vi "Sparger_syringe_rinsing_subVI_BM.vi"(4 "N syringe rinses":i32=3, 5 "COM Port":refnum<visa-resource-name>="COM12", 6 "N sparge rinses":i32=3, 7 "Pump Parameters":T1={"Speed 1"="150", "Speed 2"="250", "Speed 3"="450", "Speed 4"="250", "UW/Sample"="5", "Sparge"="2", "Std"="4", "Waste"="15", "Air"="14", "Milli-Q"="1", "H2SO4"="6", "NaOH"="3", "Catalyst"="7", "Cell (H+ side)"="8", "Cell (sample side)"="9", "NaCl"="11"}, 8 "Extra Milli-Q (ml)":dbl=2.0, 9 "step to ml":dbl=1920.0, 10 "Total Vol. (mL)":dbl=12.0, 11 "Sample Volume":dbl=10.0) -> ()   [LabVIEW 2021]
panel:
  out "Full Command":string="V450O1P38400O15D38400"
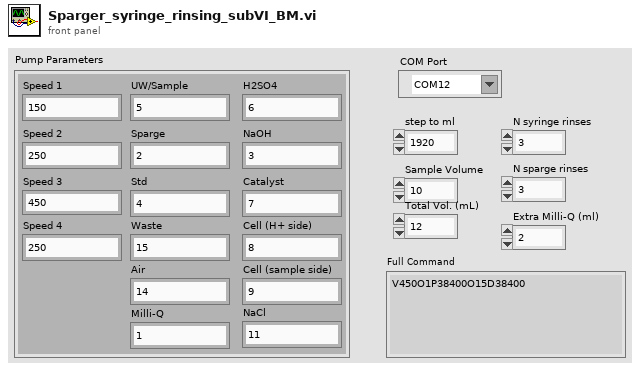
[diagram p1: front panel]
types:
  T1 = cluster{"Speed 1":string, "Speed 2":string, "Speed 3":string, "Speed 4":string, "UW/Sample":string, "Sparge":string, "Std":string, "Waste":string, "Air":string, "Milli-Q":string, "H2SO4":string, "NaOH":string, "Catalyst":string, "Cell (H+ side)":string, "Cell (sample side)":string, "NaCl":string}
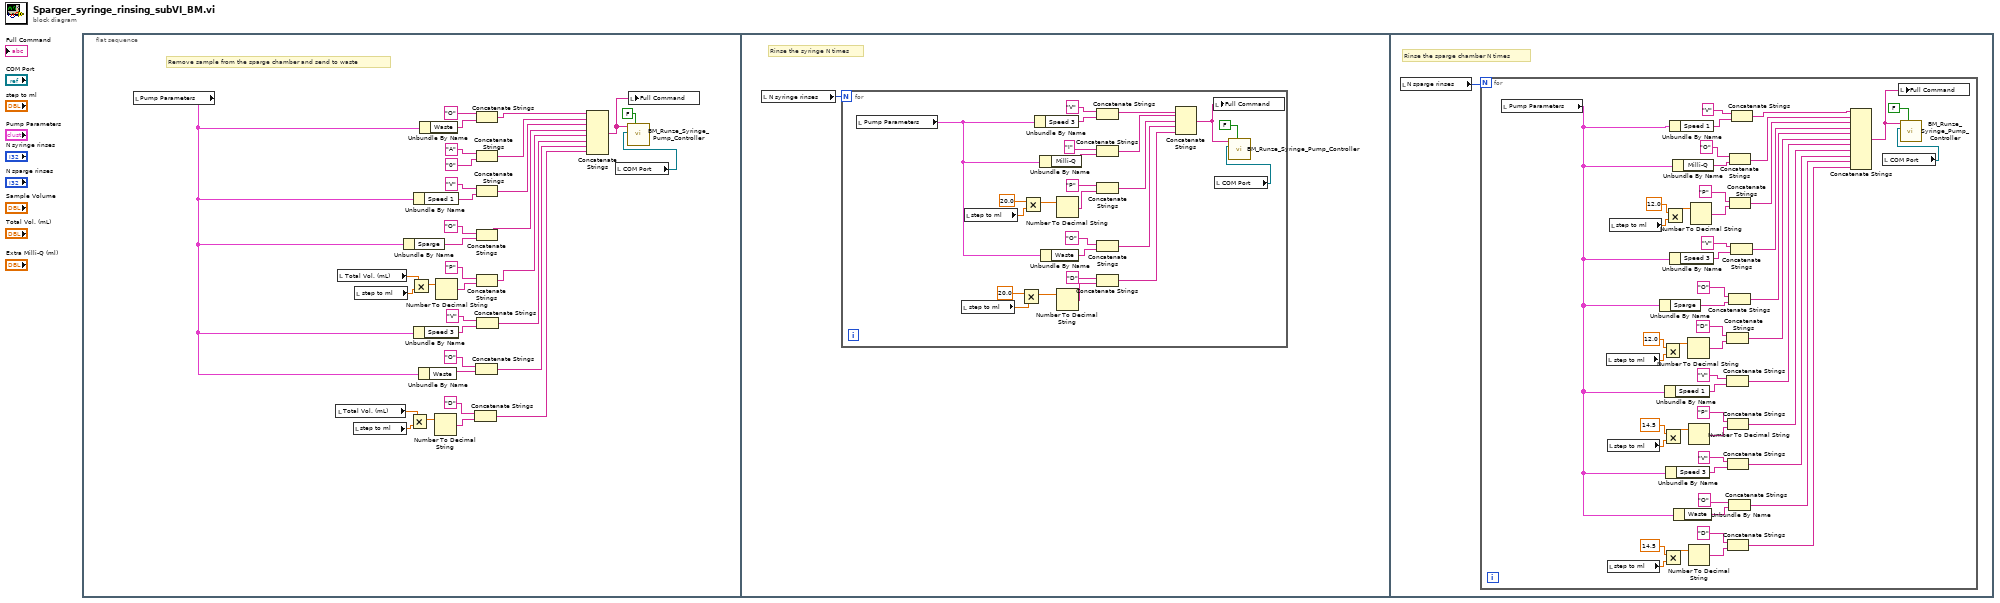
[diagram p0: block diagram]
diagram:
  n1 = flat-sequence {
    frame #0 {
      # "Remove sample from the sparge chamber and send to waste"
      n2 = local read "Pump Parameters"() -> (w16:T1)
      n3 = local read "Total Vol. (mL)"() -> (w4:dbl)
      n4 = local read "Total Vol. (mL)"() -> (w30:dbl)
      n5 = local read "step to ml"() -> (w3:dbl)
      n6 = local read "step to ml"() -> (w31:dbl)
      n7 = Unbundle By Name(w16) -> ("Sparge"=w29:string)
      n8 = Multiply(x=w4, y=w3) -> (x*y=w2:dbl)
      n9 = Multiply(x=w30, y=w31) -> (x*y=w32:dbl)
      n10 = Unbundle By Name(w16) -> ("Speed 1"=w20:string)
      n11 = Unbundle By Name(w16) -> ("Speed 3"=w19:string)
      n12 = Unbundle By Name(w16) -> ("Waste"=w21:string)
      n13 = Unbundle By Name(w16) -> ("Waste"=w33:string)
      n14 = Number To Decimal String(number=w2) -> (decimal integer string=w5:string)  [unwired: 1 out]
      n15 = Number To Decimal String(number=w32) -> (decimal integer string=w28:string)  [unwired: 1 out]
      n16 = Concatenate Strings("D", w5) -> (w1:string)
      n17 = Concatenate Strings("O", w21) -> (w17:string)
      n18 = Concatenate Strings("O", w33) -> (w27:string)
      n19 = Concatenate Strings("A", "0") -> (w26:string)
      n20 = Concatenate Strings("V", w20) -> (w25:string)
      n21 = Concatenate Strings("O", w29) -> (w24:string)
      n22 = Concatenate Strings("P", w28) -> (w23:string)
      n23 = Concatenate Strings("V", w19) -> (w18:string)
      n24 = Concatenate Strings(w27, w26, w25, w24, w23, w18, w17, w1) -> (w22:string)
      n25 = local read "COM Port"() -> (w34:refnum<visa-resource-name>)
      n26 = call "BM_Runze_Syringe_Pump_Controller.vi"("Initialize Plunger?"=FALSE ("Initialize?"), "COM Port (Runze)"=w34, "Enter Command"=w22) -> ()  [unwired: 6 in, 3 out]
      n27 = local write "Full Command"(w22) -> ()
    }
    frame #1 {
      # "Rinse the syringe N times"
      n28 = local read "N syringe rinses"() -> (w35:i32)
      n29 = for {
        N: w35 -> [_]
        n30 = local read "Pump Parameters"() -> (w42:T1)
        n31 = local read "step to ml"() -> (w43:dbl)
        n32 = local read "step to ml"() -> (w54:dbl)
        n33 = Multiply(x=20.0, y=w43) -> (x*y=w46:dbl)
        n34 = Multiply(x=20.0, y=w54) -> (x*y=w55:dbl)
        n35 = Unbundle By Name(w42) -> ("Speed 3"=w50:string)
        n36 = Unbundle By Name(w42) -> ("Milli-Q"=w57:string)
        n37 = Unbundle By Name(w42) -> ("Waste"=w48:string)
        n38 = Number To Decimal String(number=w55) -> (decimal integer string=w52:string)  [unwired: 1 out]
        n39 = Number To Decimal String(number=w46) -> (decimal integer string=w45:string)  [unwired: 1 out]
        n40 = Concatenate Strings("V", w50) -> (w41:string)
        n41 = Concatenate Strings("I", w57) -> (w40:string)
        n42 = Concatenate Strings("P" ("string"), w52) -> (w39:string)
        n43 = Concatenate Strings("O", w48) -> (w38:string)
        n44 = Concatenate Strings("D" ("string"), w45) -> (w37:string)
        n45 = Concatenate Strings(w41, w40, w39, w38, w37) -> (w58:string)
        n46 = local write "Full Command"(w58) -> ()
        n47 = local read "COM Port"() -> (w59:refnum<visa-resource-name>)
        n48 = call "BM_Runze_Syringe_Pump_Controller.vi"("Initialize Plunger?"=FALSE ("Initialize?"), "COM Port (Runze)"=w59, "Enter Command"=w58) -> ()  [unwired: 6 in, 3 out]
      }
    }
    frame #2 {
      # "Rinse the sparge chamber N times"
      n49 = local read "N sparge rinses"() -> (w61:i32)
      n50 = for {
        N: w61 -> [_]
        n51 = local read "Pump Parameters"() -> (w65:T1)
        n52 = local read "step to ml"() -> (w105:dbl)
        n53 = local read "step to ml"() -> (w102:dbl)
        n54 = local read "step to ml"() -> (w99:dbl)
        n55 = local read "step to ml"() -> (w108:dbl)
        n56 = Unbundle By Name(w65) -> ("Sparge"=w92:string)
        n57 = Multiply(x=12.0, y=w105) -> (x*y=w106:dbl)
        n58 = Multiply(x=14.5, y=w102) -> (x*y=w103:dbl)
        n59 = Multiply(x=14.5, y=w99) -> (x*y=w100:dbl)
        n60 = Multiply(x=12.0, y=w108) -> (x*y=w109:dbl)
        n61 = Unbundle By Name(w65) -> ("Speed 1"=w82:string)
        n62 = Unbundle By Name(w65) -> ("Speed 3"=w62:string)
        n63 = Unbundle By Name(w65) -> ("Speed 1"=w84:string)
        n64 = Unbundle By Name(w65) -> ("Speed 3"=w63:string)
        n65 = Unbundle By Name(w65) -> ("Milli-Q"=w96:string)
        n66 = Unbundle By Name(w65) -> ("Waste"=w68:string)
        n67 = Number To Decimal String(number=w106) -> (decimal integer string=w90:string)  [unwired: 1 out]
        n68 = Number To Decimal String(number=w103) -> (decimal integer string=w88:string)  [unwired: 1 out]
        n69 = Number To Decimal String(number=w100) -> (decimal integer string=w86:string)  [unwired: 1 out]
        n70 = Number To Decimal String(number=w109) -> (decimal integer string=w94:string)  [unwired: 1 out]
        n71 = Concatenate Strings("D", w90) -> (w75:string)
        n72 = Concatenate Strings("V", w82) -> (w74:string)
        n73 = Concatenate Strings("P", w88) -> (w73:string)
        n74 = Concatenate Strings("V", w62) -> (w72:string)
        n75 = Concatenate Strings("D", w86) -> (w66:string)
        n76 = Concatenate Strings("O", w92) -> (w76:string)
        n77 = Concatenate Strings("O", w68) -> (w67:string)
        n78 = Concatenate Strings("O", w96) -> (w79:string)
        n79 = Concatenate Strings("P", w94) -> (w78:string)
        n80 = Concatenate Strings("V", w63) -> (w77:string)
        n81 = Concatenate Strings("V", w84) -> (w80:string)
        n82 = Concatenate Strings(w80, w79, w78, w77, w76, w75, w74, w73, w72, w67, w66) -> (w70:string)
        n83 = local read "COM Port"() -> (w71:refnum<visa-resource-name>)
        n84 = local write "Full Command"(w70) -> ()
        n85 = call "BM_Runze_Syringe_Pump_Controller.vi"("Initialize Plunger?"=FALSE ("Initialize?"), "COM Port (Runze)"=w71, "Enter Command"=w70) -> ()  [unwired: 6 in, 3 out]
      }
    }
  }
